vi "Start DB Vis.vi"(8 "error in (no error)":errorcluster) -> (0 "error out":errorcluster)   [LabVIEW 2012]
panel:
  out "Front Panel Window:Open 2":bool
  out "Front Panel Window:Open":bool
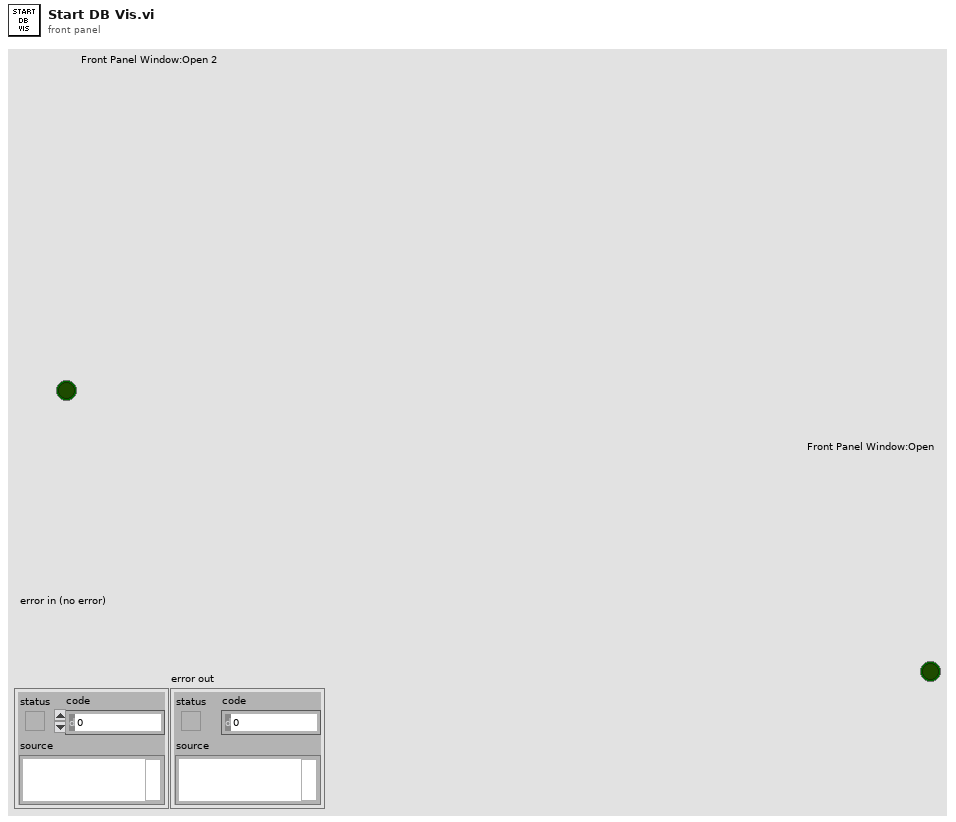
[diagram p1: front panel]
types:
  T1 = enum32{"Bad", "Idle", "Run top level", "Running"}
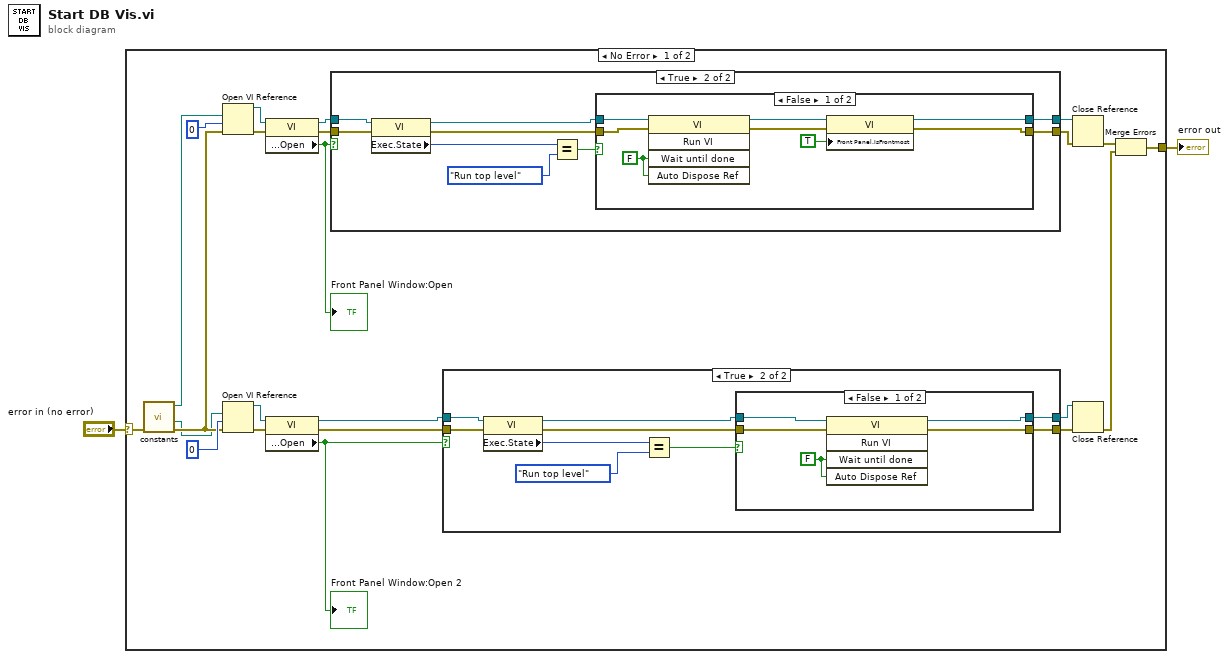
[diagram p0: block diagram]
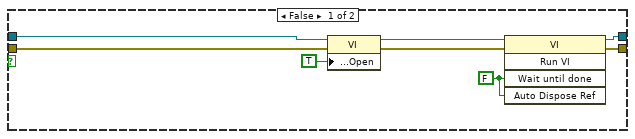
[diagram p2: hidden frame]
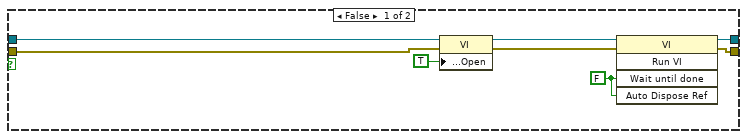
[diagram p4: hidden frame]
diagram:
  n1 = case shown="No Error" "error in (no error)" {
    selector: "error in (no error)" -> [w3 w77]
    tunnel: [w4 w77] -> w1
    frame No Error {
      n2 = call "constants.vi"("error in (no error)"=w3) -> ("error out"=w7:errorcluster, "batch updater file path"=w5:path, "DB connection File Path"=w6:path)  [unwired: 4 in, 4 out]
      n3 = Open VI Reference(vi path=w6, options=0, error in (no error)=w7) -> (vi reference=w21:refnum<vi>, error out=w23:errorcluster)  [unwired: 3 in]
      n4 = Open VI Reference(vi path=w5, options=0, error in (no error)=w7) -> (vi reference=w12:refnum<vi>, error out=w14:errorcluster)  [unwired: 3 in]
      n5 = property class="VI"(reference=w21, error in=w23) -> (reference out=w17:refnum<vi>, error out=w22:errorcluster, "Front Panel.Open"=w24:bool)
      "Front Panel Window:Open" <- w24
      n6 = property class="VI"(reference=w12, error in=w14) -> (reference out=w9:refnum<vi>, error out=w13:errorcluster, "Front Panel.Open"=w15:bool)
      "Front Panel Window:Open 2" <- w15
      n7 = case shown="True" w24 {
        tunnel: w22 -> [w57 w65]
        tunnel: [w53 w58] -> w19
        tunnel: w17 -> [w52 w66]
        tunnel: [w54 w59] -> w25
        frame False {
          w50 = FALSE ("Wait Until Done")
          n8 = property class="VI"(reference=w52, error in=w57, "Front Panel.Open"=TRUE ("Front Panel Window:Open")) -> (reference out=w56:refnum<vi>, error out=w55:errorcluster)
          n9 = invoke class="VI" method="Run VI"(reference=w56, error in=w55, "Wait until done"=w50, "Auto Dispose Ref"=w50) -> (reference out=w54:refnum<vi>, error out=w53:errorcluster)  [unwired: 1 in, 3 out]
        }
        frame True {
          n10 = property class="VI"(reference=w66, error in=w65) -> (reference out=w61:refnum<vi>, error out=w60:errorcluster, "Exec.State"=w64:T1)
          n11 = Equal?(x=w64, y=T1."Run top level" ("Execution:State 2")) -> (x = y?=w62:bool)
          n12 = case shown="False" w62 {
            tunnel: w61 -> [w73 w76]
            tunnel: w60 -> [w72 w75]
            tunnel: [w69 w76] -> w59
            tunnel: [w68 w75] -> w58
            frame False {
              w74 = FALSE ("Wait Until Done")
              n13 = invoke class="VI" method="Run VI"(reference=w73, error in=w72, "Wait until done"=w74, "Auto Dispose Ref"=w74) -> (reference out=w71:refnum<vi>, error out=w70:errorcluster)  [unwired: 1 in, 3 out]
              n14 = property class="VI"(reference=w71, error in=w70, "Front Panel.IsFrontmost"=TRUE ("Front Panel Window:Is Frontmost")) -> (reference out=w69:refnum<vi>, error out=w68:errorcluster)
            }
            frame True {
            }
          }
        }
      }
      n15 = case shown="True" w15 {
        tunnel: w13 -> [w33 w41]
        tunnel: [w29 w34] -> w10
        tunnel: w9 -> [w28 w42]
        tunnel: [w30 w35] -> w16
        frame False {
          w26 = FALSE ("Wait Until Done")
          n16 = property class="VI"(reference=w28, error in=w33, "Front Panel.Open"=TRUE ("Front Panel Window:Open")) -> (reference out=w32:refnum<vi>, error out=w31:errorcluster)
          n17 = invoke class="VI" method="Run VI"(reference=w32, error in=w31, "Wait until done"=w26, "Auto Dispose Ref"=w26) -> (reference out=w30:refnum<vi>, error out=w29:errorcluster)  [unwired: 1 in, 3 out]
        }
        frame True {
          n18 = property class="VI"(reference=w42, error in=w41) -> (reference out=w37:refnum<vi>, error out=w36:errorcluster, "Exec.State"=w40:T1)
          n19 = Equal?(x=w40, y=T1."Run top level" ("Execution:State 2")) -> (x = y?=w38:bool)
          n20 = case shown="False" w38 {
            tunnel: w37 -> [w46 w49]
            tunnel: w36 -> [w45 w48]
            tunnel: [w44 w49] -> w35
            tunnel: [w43 w48] -> w34
            frame False {
              w47 = FALSE ("Wait Until Done")
              n21 = invoke class="VI" method="Run VI"(reference=w46, error in=w45, "Wait until done"=w47, "Auto Dispose Ref"=w47) -> (reference out=w44:refnum<vi>, error out=w43:errorcluster)  [unwired: 1 in, 3 out]
            }
            frame True {
            }
          }
        }
      }
      n22 = Close Reference(reference=w25, error in (no error)=w19) -> (error out=w18:errorcluster)
      n23 = Close Reference(reference=w16, error in (no error)=w10) -> (error out=w8:errorcluster)
      n24 = Merge Errors(w18, w8) -> (w4:errorcluster)
    }
    frame Error {
    }
  }
  "error out" <- w1
